vi "Stages Messenger.vi"(0 "Stage Notifier Name":string, 2 "Actions":T2, 5 "Setpoint":dbl[](array[numeric]), 7 "Axis":bool[](array[boolean]), 9 "Velocity":dbl, 11 "Misc":variant, 13 "Exit While Busy?":bool) -> (4 "Stage Notifier Name (Dup)":string, 6 "Positions":dbl[](array[numeric]), 8 "Status":T1, 10 "Velocity Out":dbl, 15 "Error":errorcluster)   [LabVIEW 2020]
uses:
  Stages Controls/Stage Actions.ctl
  Stages Controls/Stage Status.ctl
  Stages Controls/Stage Notifier Element.ctl
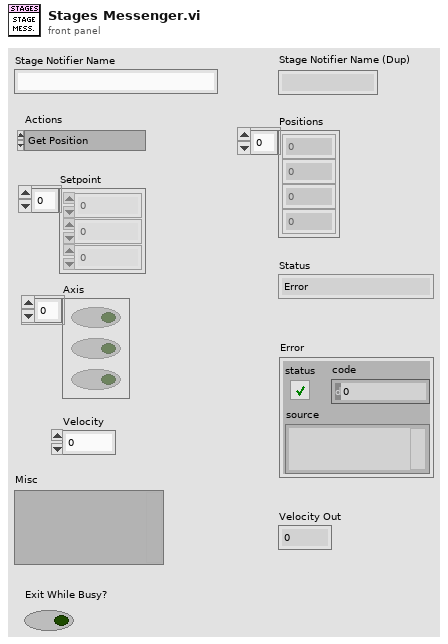
[diagram p1: front panel]
types:
  T1 = typedef "Stage Status.ctl" = enum16{"Error", "Abort", "Busy", "On Target"}
  T2 = typedef "Stage Actions.ctl" = enum16{"Get Position", "MVR", "MOVE", "HALT", "ONTARGET", "ERROR", "REFERENCE", "INIT", "VELOCITY", "STATUS", "EXIT", "HOME", "ZEROPOS", "NANOPOS", "ANALOG", "QUIT"}
  T3 = typedef "Stage Notifier Element.ctl" = cluster{"Action":T2, "Axis":bool[], "Setpoint":dbl[], "Velocity":dbl, "Cmd Recvd?":bool, "Position":dbl[], "Status":T1, "Misc":variant}
  T4 = typedef "Stage Limits.ctl" = cluster{"Notifier":string, "Use Limits":bool, "Limits":dbl[][]}
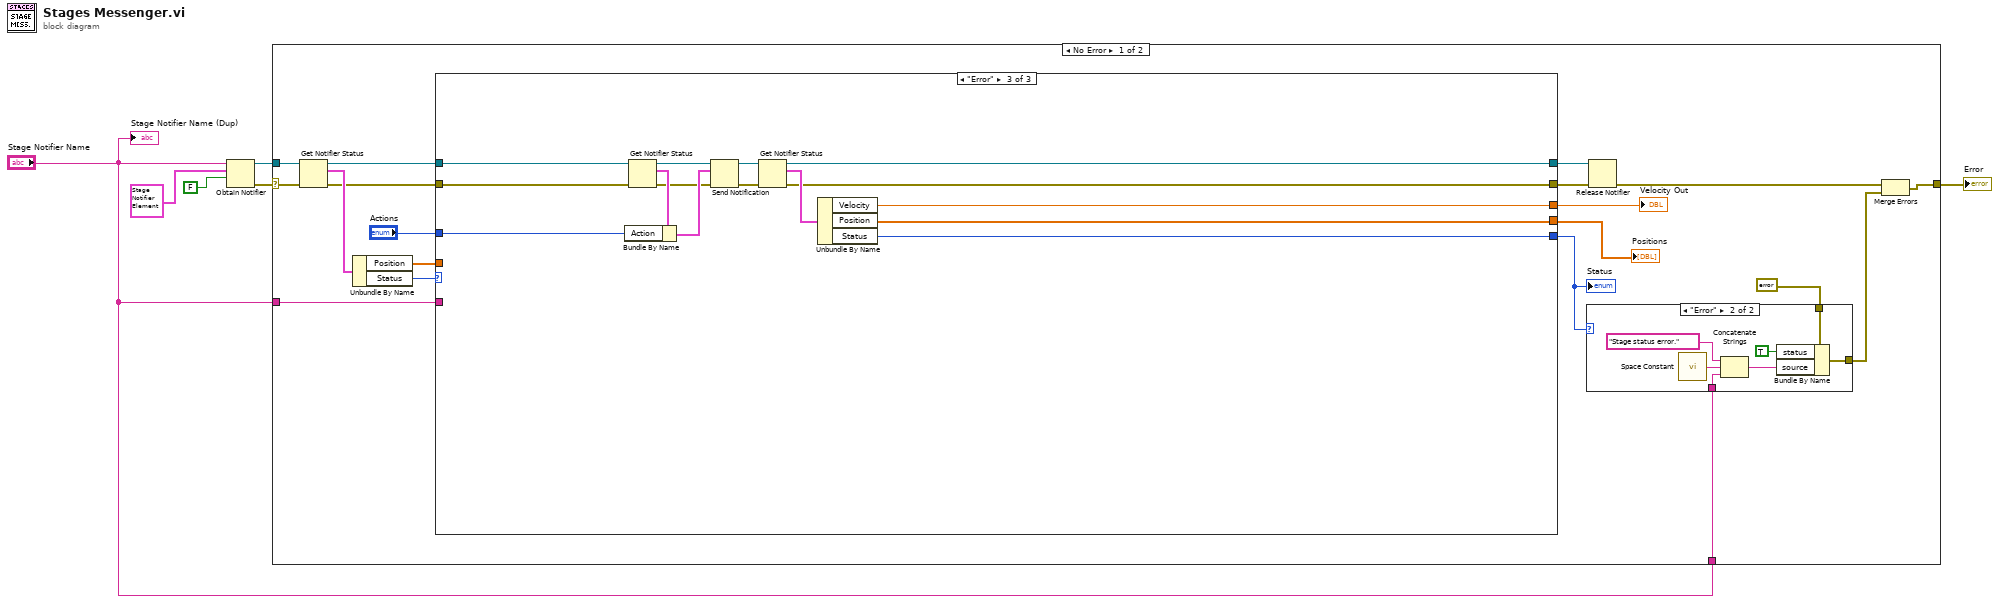
[diagram p0: block diagram]
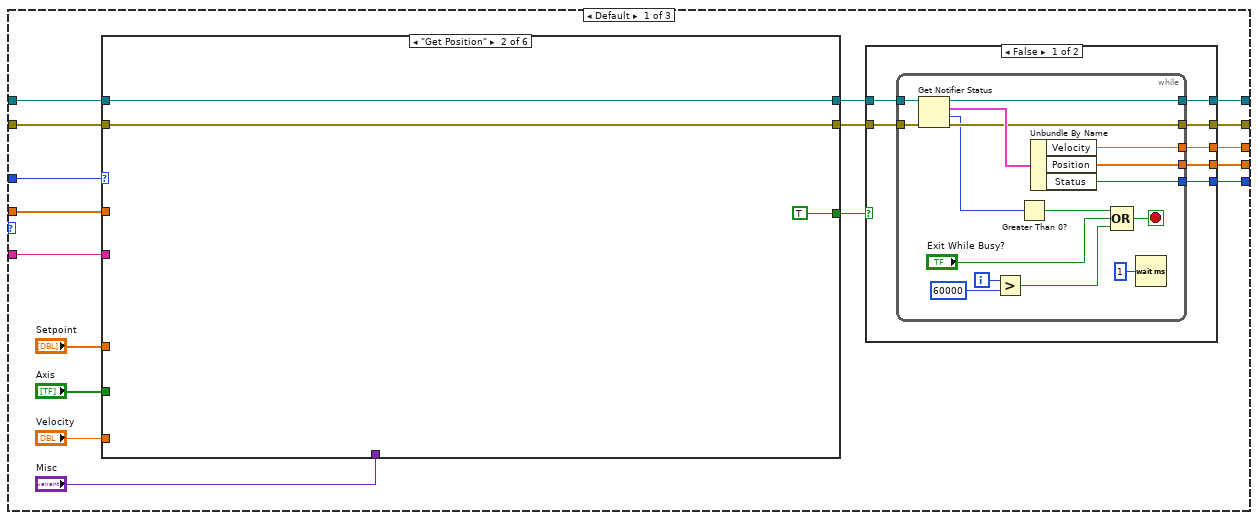
[diagram p3: hidden frame]
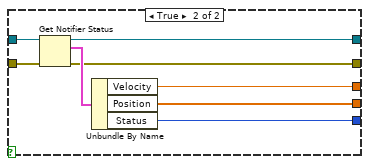
[diagram p4: hidden frame]
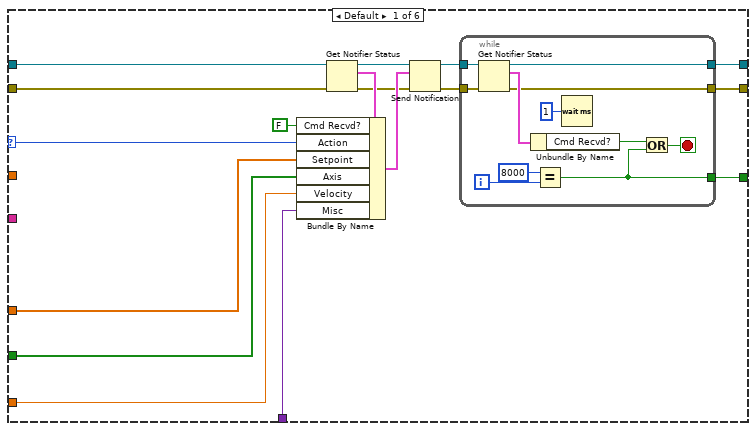
[diagram p5: hidden frame]
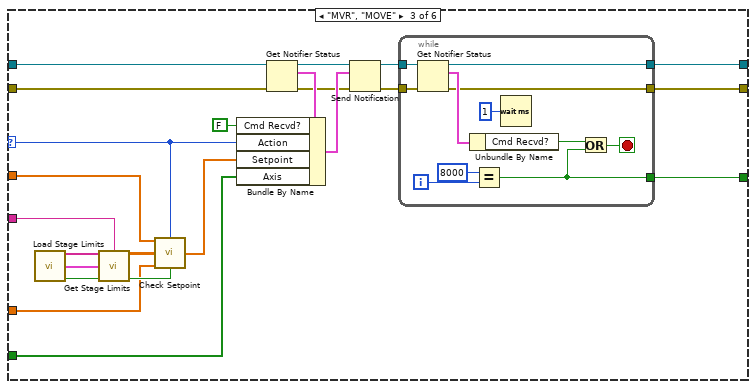
[diagram p6: hidden frame]
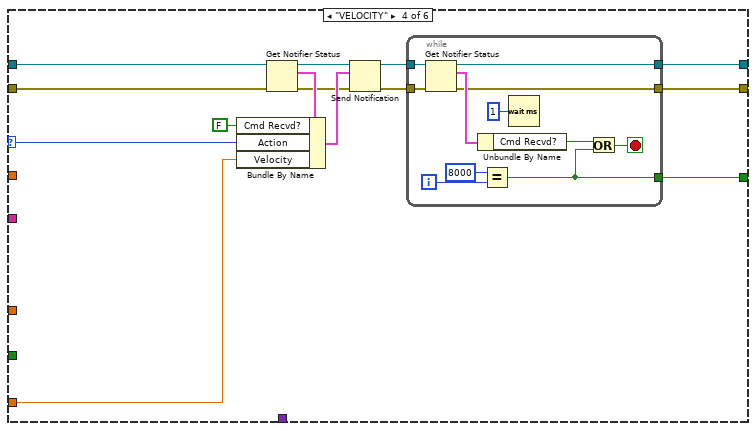
[diagram p7: hidden frame]
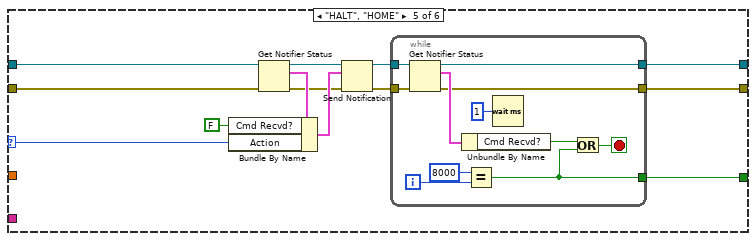
[diagram p8: hidden frame]
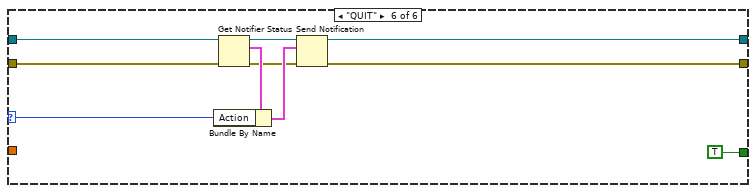
[diagram p9: hidden frame]
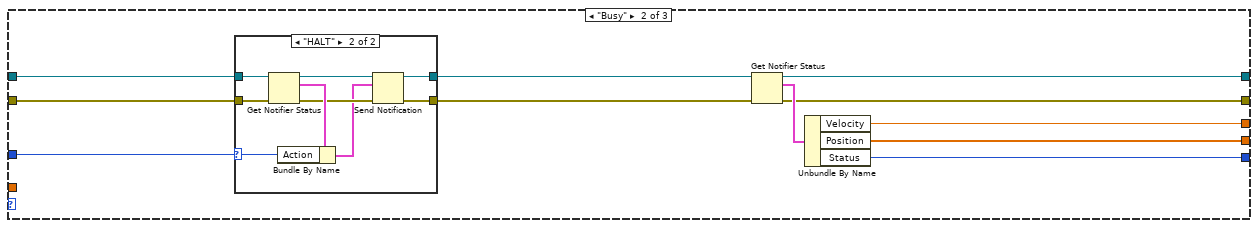
[diagram p10: hidden frame]
diagram:
  n1 = Obtain Notifier(name (unnamed)="Stage Notifier Name", notification data type=T3 {"Action"=enum."Get Position", "Axis"=[], "Setpoint"=[], "Velocity"=0.5, "Cmd Recvd?"=FALSE, "Position"=[], "Status"=enum."Error", "Misc"=variant} ("Stage Status"), create if not found? (T)=FALSE) -> (notifier out=w3:refnum<notifier>, error out=w4:errorcluster)  [unwired: 1 in, 1 out]
  n2 = case shown="No Error" w4 {
    selector: w4 -> [w19 w243]
    tunnel: w3 -> [w25 _]
    tunnel: "Stage Notifier Name" -> [w14 _]
    tunnel: [w11 w243] -> w2
    tunnel: "Stage Notifier Name" -> [w8 _]
    frame No Error {
      n3 = Get Notifier Status(notifier=w25, error in (no error)=w19) -> (notifier out=w23:refnum<notifier>, current notification=w24:T3, error out=w18:errorcluster)  [unwired: 2 out]
      n4 = Unbundle By Name(w24) -> ("Position"=w9:dbl[], "Status"=w16:T1)
      n5 = case shown="\"Error\"" w16 {
        tunnel: w23 -> [w50 w210 w242]
        tunnel: [w43 w215 w236] -> w22
        tunnel: [w42 w214 w235] -> w21
        tunnel: [w41 w213 w234] -> w15
        tunnel: "Actions" -> [w49 w211 w240]
        tunnel: w18 -> [w40 w209 w232]
        tunnel: [w38 w212 w229] -> w17
        tunnel: w9 -> [w36 _ _]
        tunnel: w8 -> [w35 _ _]
        tunnel: [w34 w206 w228] -> w7
        frame Default {
          n6 = case shown="\"Get Position\"" w49 {
            selector: w49 -> [w94 _ w117 w156 w180 w201]
            tunnel: w50 -> [w95 w112 w132 w157 w181 w204]
            tunnel: [w87 w112 w128 w153 w177 w205] -> w44
            tunnel: "Setpoint" -> [w91 _ w115 _ _ _]
            tunnel: "Axis" -> [w90 _ w129 _ _ _]
            tunnel: "Velocity" -> [w89 _ _ w147 _ _]
            tunnel: "Misc" -> [w88 _ _ _ _ _]
            tunnel: [w86 TRUE w127 w152 w176 TRUE] -> w45
            tunnel: w40 -> [w85 w111 w126 w151 w175 w198]
            tunnel: [w82 w111 w123 w148 w172 w196] -> w39
            tunnel: w36 -> [_ _ w114 _ _ _]
            tunnel: w35 -> [_ _ w122 _ _ _]
            frame Default {
              n7 = Get Notifier Status(notifier=w95, error in (no error)=w85) -> (notifier out=w96:refnum<notifier>, current notification=w97:T3, error out=w84:errorcluster)  [unwired: 2 out]
              n8 = Bundle By Name(cluster=w97, "Cmd Recvd?"=FALSE, "Action"=w94, "Setpoint"=w91, "Axis"=w90, "Velocity"=w89, "Misc"=w88) -> (w98:T3)
              n9 = Send Notification(notification=w98, notifier=w96, error in (no error)=w84) -> (notifier out=w92:refnum<notifier>, error out=w83:errorcluster)
              n10 = while {
                tunnel: w92 -> [w109]
                tunnel: [w106] -> w87
                tunnel: [w102] -> w86
                tunnel: w83 -> [w100]
                tunnel: [w99] -> w82
                i -> [w105]
                stop <- w101 stop-if-true
                n11 = Get Notifier Status(notifier=w109, error in (no error)=w100) -> (notifier out=w106:refnum<notifier>, current notification=w108:T3, error out=w99:errorcluster)  [unwired: 2 out]
                n12 = Unbundle By Name(w108) -> ("Cmd Recvd?"=w103:bool)
                n13 = Equal?(x=8000, y=w105) -> (x = y?=w102:bool)
                n14 = Wait (ms)(milliseconds to wait=u32 1) -> ()  [unwired: 1 out]
                n15 = Or(x=w103, y=w102) -> (x .or. y?=w101:bool)
              }
            }
            frame "Get Position" {
            }
            frame "MVR", "MOVE" {
              n16 = call "Load Stage Limits.vi"() -> ("Notifier Names"=w119:string[], "Stage Limits"=w120:T4[], "Loaded"=w121:bool)  [unwired: 13 in]
              n17 = call "Get Stage Limits.vi"("Notifier Names"=w119, "Notifier Name"=w122, "Stage Limits"=w120, "Limits Loaded?"=w121) -> ("Limits"=w116:dbl[][], "Use Limits?"=w118:bool)  [unwired: 10 in]
              n18 = call "Check Setpoint.vi"("Positions"=w114, "Actions"=w117, "Limits"=w116, "Setpoints"=w115, "Use Limits"=w118) -> ("Setpoints Out"=w113:dbl[])  [unwired: 10 in]
              n19 = Get Notifier Status(notifier=w132, error in (no error)=w126) -> (notifier out=w133:refnum<notifier>, current notification=w134:T3, error out=w125:errorcluster)  [unwired: 2 out]
              n20 = Bundle By Name(cluster=w134, "Cmd Recvd?"=FALSE, "Action"=w117, "Setpoint"=w113, "Axis"=w129) -> (w135:T3)
              n21 = Send Notification(notification=w135, notifier=w133, error in (no error)=w125) -> (notifier out=w130:refnum<notifier>, error out=w124:errorcluster)
              n22 = while {
                tunnel: w130 -> [w146]
                tunnel: [w143] -> w128
                tunnel: [w139] -> w127
                tunnel: w124 -> [w137]
                tunnel: [w136] -> w123
                i -> [w142]
                stop <- w138 stop-if-true
                n23 = Get Notifier Status(notifier=w146, error in (no error)=w137) -> (notifier out=w143:refnum<notifier>, current notification=w145:T3, error out=w136:errorcluster)  [unwired: 2 out]
                n24 = Unbundle By Name(w145) -> ("Cmd Recvd?"=w140:bool)
                n25 = Equal?(x=8000, y=w142) -> (x = y?=w139:bool)
                n26 = Wait (ms)(milliseconds to wait=u32 1) -> ()  [unwired: 1 out]
                n27 = Or(x=w140, y=w139) -> (x .or. y?=w138:bool)
              }
            }
            frame "VELOCITY" {
              n28 = Get Notifier Status(notifier=w157, error in (no error)=w151) -> (notifier out=w158:refnum<notifier>, current notification=w159:T3, error out=w150:errorcluster)  [unwired: 2 out]
              n29 = Bundle By Name(cluster=w159, "Cmd Recvd?"=FALSE, "Action"=w156, "Velocity"=w147) -> (w160:T3)
              n30 = Send Notification(notification=w160, notifier=w158, error in (no error)=w150) -> (notifier out=w154:refnum<notifier>, error out=w149:errorcluster)
              n31 = while {
                tunnel: w154 -> [w171]
                tunnel: [w168] -> w153
                tunnel: [w164] -> w152
                tunnel: w149 -> [w162]
                tunnel: [w161] -> w148
                i -> [w167]
                stop <- w163 stop-if-true
                n32 = Get Notifier Status(notifier=w171, error in (no error)=w162) -> (notifier out=w168:refnum<notifier>, current notification=w170:T3, error out=w161:errorcluster)  [unwired: 2 out]
                n33 = Unbundle By Name(w170) -> ("Cmd Recvd?"=w165:bool)
                n34 = Equal?(x=8000, y=w167) -> (x = y?=w164:bool)
                n35 = Wait (ms)(milliseconds to wait=u32 1) -> ()  [unwired: 1 out]
                n36 = Or(x=w165, y=w164) -> (x .or. y?=w163:bool)
              }
            }
            frame "HALT", "HOME" {
              n37 = Get Notifier Status(notifier=w181, error in (no error)=w175) -> (notifier out=w182:refnum<notifier>, current notification=w183:T3, error out=w174:errorcluster)  [unwired: 2 out]
              n38 = Bundle By Name(cluster=w183, "Cmd Recvd?"=FALSE, "Action"=w180) -> (w184:T3)
              n39 = Send Notification(notification=w184, notifier=w182, error in (no error)=w174) -> (notifier out=w178:refnum<notifier>, error out=w173:errorcluster)
              n40 = while {
                tunnel: w178 -> [w195]
                tunnel: [w192] -> w177
                tunnel: [w188] -> w176
                tunnel: w173 -> [w186]
                tunnel: [w185] -> w172
                i -> [w191]
                stop <- w187 stop-if-true
                n41 = Get Notifier Status(notifier=w195, error in (no error)=w186) -> (notifier out=w192:refnum<notifier>, current notification=w194:T3, error out=w185:errorcluster)  [unwired: 2 out]
                n42 = Unbundle By Name(w194) -> ("Cmd Recvd?"=w189:bool)
                n43 = Equal?(x=8000, y=w191) -> (x = y?=w188:bool)
                n44 = Wait (ms)(milliseconds to wait=u32 1) -> ()  [unwired: 1 out]
                n45 = Or(x=w189, y=w188) -> (x .or. y?=w187:bool)
              }
            }
            frame "QUIT" {
              n46 = Get Notifier Status(notifier=w204, error in (no error)=w198) -> (notifier out=w203:refnum<notifier>, current notification=w202:T3, error out=w197:errorcluster)  [unwired: 2 out]
              n47 = Bundle By Name(cluster=w202, "Action"=w201) -> (w200:T3)
              n48 = Send Notification(notification=w200, notifier=w203, error in (no error)=w197) -> (notifier out=w205:refnum<notifier>, error out=w196:errorcluster)
            }
          }
          n49 = case shown="False" w45 {
            tunnel: w44 -> [w57 w81]
            tunnel: [w56 w80] -> w43
            tunnel: [w55 w79] -> w42
            tunnel: [w54 w77] -> w41
            tunnel: w39 -> [w53 w76]
            tunnel: [w52 w75] -> w38
            tunnel: [w51 w74] -> w34
            frame False {
              n50 = while {
                tunnel: w57 -> [w73]
                tunnel: [w72] -> w56
                tunnel: [w70] -> w55
                tunnel: [w66] -> w54
                tunnel: w53 -> [w62]
                tunnel: [w61] -> w52
                tunnel: [w58] -> w51
                i -> [w68]
                stop <- w63 stop-if-true
                n51 = Get Notifier Status(notifier=w73, error in (no error)=w62) -> (notifier out=w72:refnum<notifier>, current notification=w71:T3, # waiting=w60:i32, error out=w61:errorcluster)  [unwired: 1 out]
                n52 = Greater?(x=w68, y=60000) -> (0:w64:bool)
                n53 = Greater Than 0?(x=w60) -> (x > 0?=w59:bool)
                n54 = Unbundle By Name(w71) -> ("Velocity"=w58:dbl, "Position"=w70:dbl[], "Status"=w66:T1)
                n55 = Compound Arithmetic op=OR(w59, "Exit While Busy?", w64) -> (w63:bool)
                n56 = Wait (ms)(milliseconds to wait=u32 1) -> ()  [unwired: 1 out]
              }
            }
            frame True {
              n57 = Get Notifier Status(notifier=w81, error in (no error)=w76) -> (notifier out=w80:refnum<notifier>, current notification=w78:T3, error out=w75:errorcluster)  [unwired: 2 out]
              n58 = Unbundle By Name(w78) -> ("Velocity"=w74:dbl, "Position"=w79:dbl[], "Status"=w77:T1)
            }
          }
        }
        frame "Busy" {
          n59 = case shown="\"HALT\"" w211 {
            selector: w211 -> [_ w224]
            tunnel: w210 -> [w218 w227]
            tunnel: w209 -> [w217 w226]
            tunnel: [w218 w221] -> w208
            tunnel: [w217 w220] -> w207
            frame Default {
            }
            frame "HALT" {
              n60 = Get Notifier Status(notifier=w227, error in (no error)=w226) -> (notifier out=w223:refnum<notifier>, current notification=w225:T3, error out=w222:errorcluster)  [unwired: 2 out]
              n61 = Bundle By Name(cluster=w225, "Action"=w224) -> (w219:T3)
              n62 = Send Notification(notification=w219, notifier=w223, error in (no error)=w222) -> (notifier out=w221:refnum<notifier>, error out=w220:errorcluster)
            }
          }
          n63 = Get Notifier Status(notifier=w208, error in (no error)=w207) -> (notifier out=w215:refnum<notifier>, current notification=w216:T3, error out=w212:errorcluster)  [unwired: 2 out]
          n64 = Unbundle By Name(w216) -> ("Velocity"=w206:dbl, "Position"=w214:dbl[], "Status"=w213:T1)
        }
        frame "Error" {
          n65 = Get Notifier Status(notifier=w242, error in (no error)=w232) -> (notifier out=w239:refnum<notifier>, current notification=w241:T3, error out=w231:errorcluster)  [unwired: 2 out]
          n66 = Bundle By Name(cluster=w241, "Action"=w240) -> (w238:T3)
          n67 = Send Notification(notification=w238, notifier=w239, error in (no error)=w231) -> (notifier out=w237:refnum<notifier>, error out=w230:errorcluster)
          n68 = Get Notifier Status(notifier=w237, error in (no error)=w230) -> (notifier out=w236:refnum<notifier>, current notification=w233:T3, error out=w229:errorcluster)  [unwired: 2 out]
          n69 = Unbundle By Name(w233) -> ("Velocity"=w228:dbl, "Position"=w235:dbl[], "Status"=w234:T1)
        }
      }
      "Positions" <- w21
      "Status" <- w15
      "Velocity Out" <- w7
      n70 = case shown="\"Error\"" w15 {
        tunnel: w14 -> [_ w30]
        tunnel: [w26 w28] -> w12
        tunnel: errorcluster {"status"=FALSE, "code"=0, "source"=""} ("Error 2") -> [w26 w27]
        frame Default {
        }
        frame "Error" {
          n71 = call <vilib>:"Space Constant.vi"() -> ("String"=w31:string)
          n72 = Concatenate Strings("Stage status error." ("source"), w31, w30) -> (w29:string)
          n73 = Bundle By Name(cluster=w27, "status"=TRUE, "source"=w29) -> (w28:errorcluster)
        }
      }
      n74 = Release Notifier(notifier=w22, error in (no error)=w17) -> (error out=w13:errorcluster)  [unwired: 1 in, 2 out]
      n75 = Merge Errors(w13, w12) -> (w11:errorcluster)
    }
    frame Error {
    }
  }
  "Error" <- w2
  "Stage Notifier Name (Dup)" <- "Stage Notifier Name"
